vi "Change User Interface.vi"(8 "error in (no error)":errorcluster, 10 "User Interface.lvclass":refnum<class "UI.lvclass">, 11 "Test Step Controller in":refnum<class "Controller.lvclass">) -> (0 "error out":errorcluster, 3 "Test Step Controller out":refnum<class "Controller.lvclass">)   [LabVIEW 2016, in "Controller Actor.lvlib" / "Controller.lvclass"]
uses:
  <userlib>/Common Components/Controller/Controller.lvclass
  <userlib>/Common Components/User Interface/UI.lvclass
  <vilib>/ActorFramework/Message Enqueuer/Message Enqueuer.lvclass/Message Enqueuer.ctl
  <vilib>/ActorFramework/Message Enqueuer/Enqueue.vi
  <vilib>/ActorFramework/Stop Msg/Stop Msg.lvclass
  C:/Program Files (x86)/National Instruments/LabVIEW 2016/vi.lib/ActorFramework/Message/Message.lvclass
  <vilib>/ActorFramework/Message Priority Queue/Priority Enqueue.vi
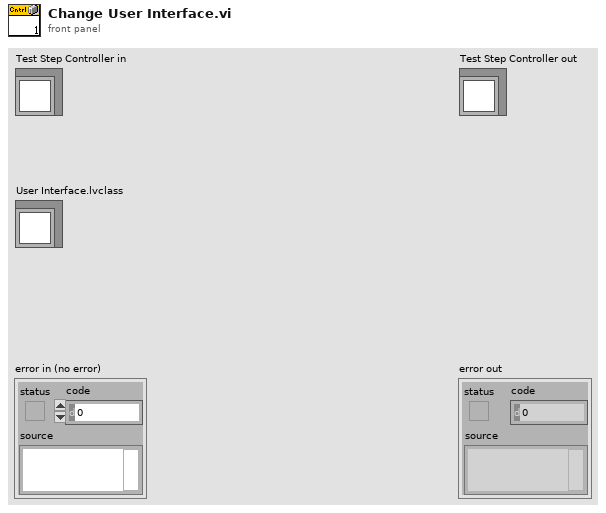
[diagram p1: front panel]
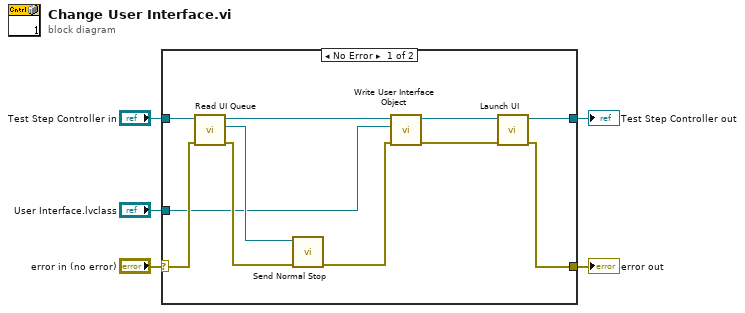
[diagram p0: block diagram]
diagram:
  n1 = case shown="No Error" "error in (no error)" {
    selector: "error in (no error)" -> [w13 w18]
    tunnel: [w15 w18] -> w4
    tunnel: [w16 w17] -> w2
    tunnel: "Test Step Controller in" -> [w14 w17]
    tunnel: "User Interface.lvclass" -> [w6 _]
    frame No Error {
      n2 = call <userlib>:"Read UI Queue.vi"("error in (no error)"=w13, "UI Controller in"=w14) -> ("error out"=w11:errorcluster, "UI Queue"=w12:refnum<class "Message Enqueuer.lvclass">, "UI Controller out"=w8:refnum<class "Controller.lvclass">)  [unwired: 7 in]
      n3 = call <vilib>:"Send Normal Stop.vi"("error in (no error)"=w11, "Message Enqueuer"=w12) -> ("error out"=w10:errorcluster)  [unwired: 9 in]
      n4 = call <userlib>:"Write User Interface Object.vi"("error in (no error)"=w10, "UI.lvclass"=w6, "UI Controller in"=w8) -> ("error out"=w9:errorcluster, "UI Controller out"=w7:refnum<class "Controller.lvclass">)  [unwired: 7 in]
      n5 = call-dynamic "Launch UI.vi"("error in (no error)"=w9, "UI Controller in"=w7) -> ("error out"=w15:errorcluster, "UI Controller out"=w16:refnum<class "Controller.lvclass">)  [unwired: 8 in]
    }
    frame Error {
    }
  }
  "error out" <- w4
  "Test Step Controller out" <- w2
